vi "Set Batch Controls.vi"(8 "error in (no error)":errorcluster, 9 "Indicator Values":variant[](array[variant]), 10 "Indicator Names":string[](array[string]), 11 "Controls_Mgr in":refnum<class "Controls_Mgr.lvclass">) -> (0 "error out":errorcluster, 3 "Controls_Mgr out":refnum<class "Controls_Mgr.lvclass">)   [LabVIEW 2015, in "Generic Module Library.lvlib" / "Template G_Module.lvlib" / "Controls_Mgr.lvclass"]
uses:
  Controls_Mgr.lvclass
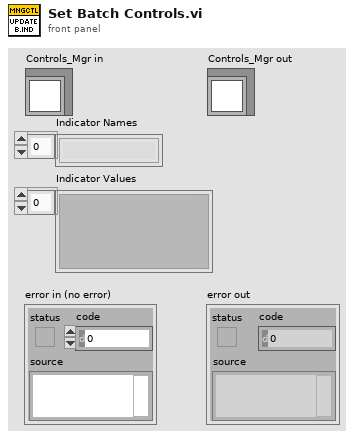
[diagram p1: front panel]
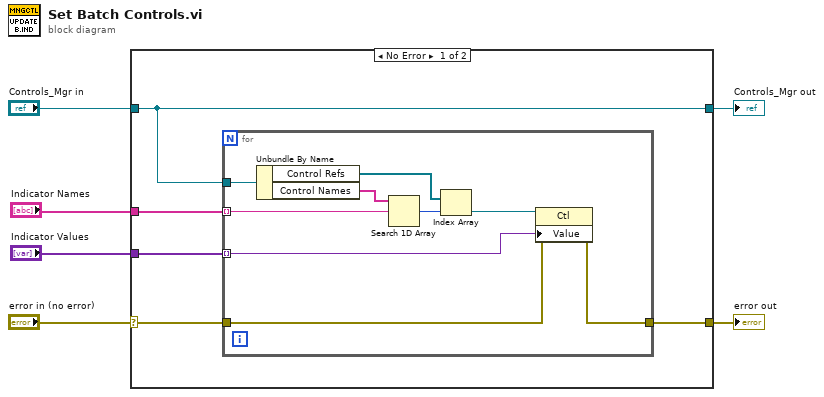
[diagram p0: block diagram]
diagram:
  n1 = case shown="No Error" "error in (no error)" {
    selector: "error in (no error)" -> [w11 w22]
    tunnel: [w7 w22] -> w5
    tunnel: [w9 w21] -> w3
    tunnel: "Controls_Mgr in" -> [w9 w21]
    tunnel: "Indicator Values" -> [w8 _]
    tunnel: "Indicator Names" -> [w10 _]
    frame No Error {
      n2 = for {
        tunnel: w10 -> [w20] mode=indexing
        tunnel: w9 -> [w19]
        tunnel: w8 -> [w13] mode=indexing
        tunnel: w11 -> [w12]
        tunnel: [w14] -> w7
        n3 = Unbundle By Name(w19) -> ("Control Refs"=w16:refnum<vi>[], "Control Names"=w18:string[])
        n4 = Search 1D Array(1D array=w18, element=w20) -> (index of element=w17:i32)  [unwired: 1 in]
        n5 = Index Array(array=w16, index=w17) -> (element=w15:refnum<vi>)
        n6 = property class="Ctl"(reference=w15, error in=w12, "Value"=w13) -> (error out=w14:errorcluster)  [unwired: 1 out]
      }
    }
    frame Error {
    }
  }
  "error out" <- w5
  "Controls_Mgr out" <- w3
